vi "Get PV.vi"(11 "Stand in":refnum<class "Stand.lvclass">) -> (2 "Stat Data.scl mean":dbl)   [LabVIEW 2019, in "Stand.lvclass"]
uses:
  Stand.lvclass
  AI_class/AI.lvclass
  FPGA/TypeDef/AI index.ctl
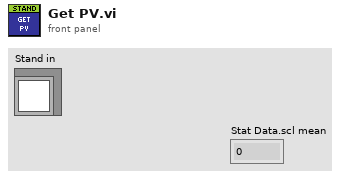
[diagram p1: front panel]
types:
  T1 = typedef "Pressure PV  Source.ctl" = enum16{"AI 5 HPP", "AI 6 DUT", "AI 7 CHMBR", "MB DUT", "MB CHMBR"}
  T2 = typedef "AI index.ctl" = u8
  T3 = typedef "AI_Data.ctl" = cluster{"Stat Data":T4, "OutOfRangeMax":bool, "OutOfRangeMin":bool, "HIHI":bool, "HI":bool, "LO":bool, "LOLO":bool, "DATA N":T5, "DATA PERIOD":T5, "UPPER TH":dbl, "LOWER TH":dbl}
  T4 = typedef "AI Statistics Data.ctl" = cluster{"raw mean":dbl, "scl mean":dbl, "raw mean 1Hz":dbl, "scl mean 1Hz":dbl}
  T5 = typedef "DATA Oscill.ctl" = cluster{"SUM":dbl, "COUNTER":dbl, "MAX CURR":dbl, "MIN CURR":dbl, "AVR":dbl, "MAX":dbl, "MIN":dbl, "DELTA AVR":dbl, "DELTA MAX":dbl, "DELTA MIN":dbl, "PERIOD":dbl}
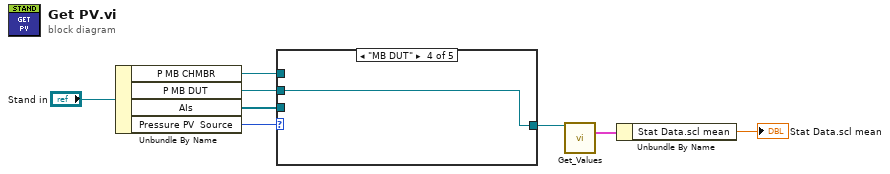
[diagram p0: block diagram]
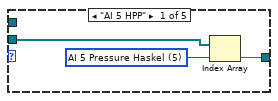
[diagram p2: hidden frame]
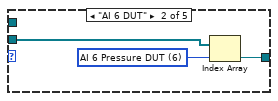
[diagram p3: hidden frame]
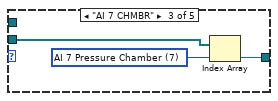
[diagram p4: hidden frame]
diagram:
  n1 = Unbundle By Name("Stand in") -> ("P MB CHMBR"=w1:refnum<class "AI.lvclass">, "P MB DUT"=w2:refnum<class "AI.lvclass">, "AIs"=w4:refnum<class "AI.lvclass">[], "Pressure PV  Source"=w6:T1)
  n2 = case shown="\"MB DUT\"" w6 {
    tunnel: w4 -> [w11 w14 w17 _ _]
    tunnel: [w9 w12 w15 w18 w19] -> w3
    tunnel: w2 -> [_ _ _ w18 _]
    tunnel: w1 -> [_ _ _ _ w19]
    frame "AI 5 HPP" {
      w10 = T2 5 items=["AI 0 Cooling Station Level", "AI 1 Cooling Station Temp", "AI 2 Oil Supply Level", "AI 3 Oil Supply Temp", "AI 4 ", "AI 5 Pressure Haskel", "AI 6 Pressure DUT", "AI 7 Pressure Chamber", "AI 8 Pressure Air inlet", "AI 9 Pressure Air outlet", "AI 10 Pressure Messure Line"] ("AI index")
      n3 = Index Array(array=w11, index=w10) -> (element=w9:refnum<class "AI.lvclass">)
    }
    frame "AI 6 DUT" {
      w13 = T2 6 items=["AI 0 Cooling Station Level", "AI 1 Cooling Station Temp", "AI 2 Oil Supply Level", "AI 3 Oil Supply Temp", "AI 4 ", "AI 5 Pressure Haskel", "AI 6 Pressure DUT", "AI 7 Pressure Chamber", "AI 8 Pressure Air inlet", "AI 9 Pressure Air outlet", "AI 10 Pressure Messure Line"] ("AI index")
      n4 = Index Array(array=w14, index=w13) -> (element=w12:refnum<class "AI.lvclass">)
    }
    frame "AI 7 CHMBR" {
      w16 = T2 7 items=["AI 0 Cooling Station Level", "AI 1 Cooling Station Temp", "AI 2 Oil Supply Level", "AI 3 Oil Supply Temp", "AI 4 ", "AI 5 Pressure Haskel", "AI 6 Pressure DUT", "AI 7 Pressure Chamber", "AI 8 Pressure Air inlet", "AI 9 Pressure Air outlet", "AI 10 Pressure Messure Line"] ("AI index")
      n5 = Index Array(array=w17, index=w16) -> (element=w15:refnum<class "AI.lvclass">)
    }
    frame "MB DUT" {
    }
    frame "MB CHMBR" {
    }
  }
  n6 = call "Get_Values.vi"("reference in"=w3) -> ("Data"=w7:T3)  [unwired: 14 in]
  n7 = Unbundle By Name(w7) -> ("Stat Data.scl mean"=→"Stat Data.scl mean":dbl)
